vi "checkFinishPrepareKickoffAllyPlay.vi"(8 "error in (no error)":errorcluster, 9 "last command_interpreted":T1, 10 "Game":refnum<class "Game.lvclass">, 11 "PrepareKickoffAllyPlay in":refnum<class "PrepareKickoffAllyPlay.lvclass">) -> (0 "error out":errorcluster, 2 "Boolean":bool, 3 "PrepareKickoffAllyPlay out":refnum<class "PrepareKickoffAllyPlay.lvclass">)   [LabVIEW 2023, in "PrepareKickoffAllyPlay.lvclass"]
uses:
  PrepareKickoffAllyPlay.lvclass
  Game_class/Game.lvclass
  Referee_class/command_interpreted.ctl
  Game_class/Game.lvclass/Game.ctl
  Referee_class/Referee.lvclass/Referee.ctl
  Game_class/Read Referee.vi
  Referee_class/Read command_interpreted.vi
  Referee_class/Referee.lvclass
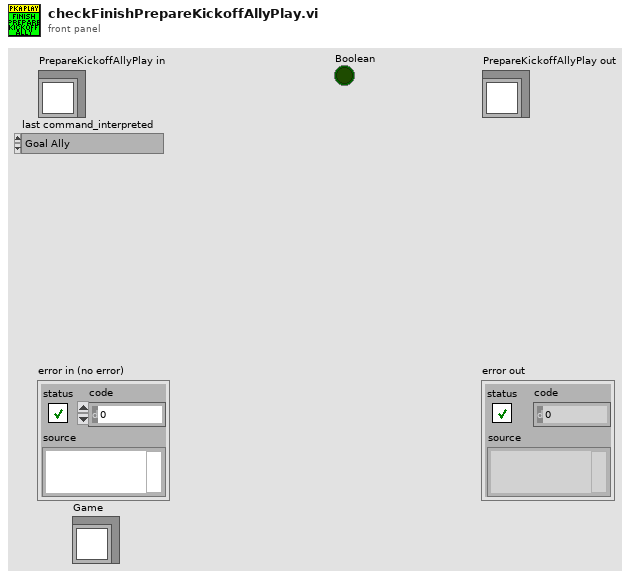
[diagram p1: front panel]
types:
  T1 = typedef "command_interpreted.ctl" = enum16{"Goal Ally", "Goal Enemy", "Ball Placement Enemy", "Ball Placement Ally", "Normal Half Time", "Extra Time  Break", "Extra Half Time", "None", "Post Game", "PKA Normal Start", "Prepare Kickoff Ally", "PKE Normal Start", "Prepare Kickoff Enemy", "Force Start", "Halt", "Timeout", "Prepare Penalty Ally", "Prepare Penalty Enemy", "PPA NormalStart", "PPE Normal Start", "Indirect Free Ally", "Direct Free Enemy", "Direct Free Ally", "Indirect Free Enemy", "Stop"}
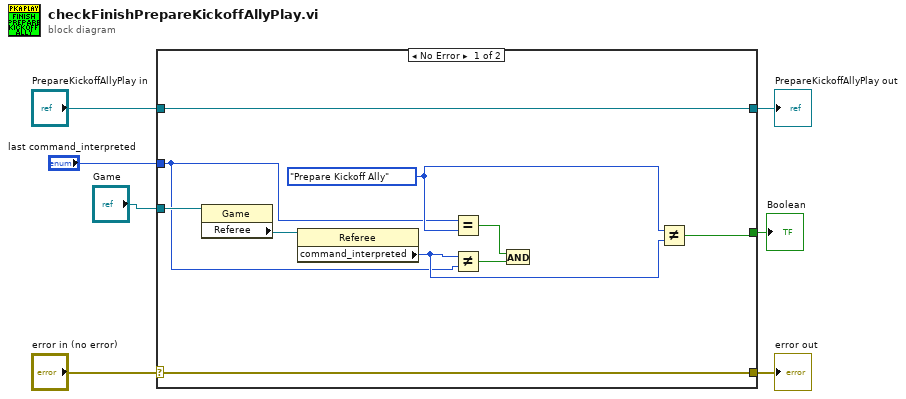
[diagram p0: block diagram]
diagram:
  n1 = case shown="No Error" "error in (no error)" {
    selector: "error in (no error)" -> [w16 w19]
    tunnel: [w16 w19] -> w6
    tunnel: [w17 w18] -> w4
    tunnel: "PrepareKickoffAllyPlay in" -> [w17 w18]
    tunnel: "Game" -> [w12 _]
    tunnel: [w11 _] -> w2
    tunnel: "last command_interpreted" -> [w8 _]
    frame No Error {
      w9 = command_interpreted."Prepare Kickoff Ally" ("command_interpreted")
      n2 = property class="Game"(reference=w12) -> ("Referee"=w15:refnum<class "Referee.lvclass">)  [unwired: 1 in, 2 out]
      n3 = property class="Referee"(reference=w15) -> ("command_interpreted"=w10:T1)  [unwired: 1 in, 2 out]
      n4 = Equal?(x=w8, y=w9) -> (x = y?=w14:bool)
      n5 = Not Equal?(x=w10, y=w8) -> (x != y?=w13:bool)
      n6 = And(x=w14, y=w13) -> ()  [unwired: 1 out]
      n7 = Not Equal?(x=w9, y=w10) -> (x != y?=w11:bool)
    }
    frame Error {
    }
  }
  "error out" <- w6
  "PrepareKickoffAllyPlay out" <- w4
  "Boolean" <- w2
